vi "PIN Verification.vi"(8 "error in (no error)":errorcluster, 10 "Array":refnum<vi>[](array[refnum]), 11 "PIN in":string) -> (0 "error out":errorcluster, 1 "Right Menu":T1, 2 "Left Menu":T1, 3 "Message Out":string, 5 "PIN":string)   [LabVIEW 2019]
uses:
  controls/Read & Write File.ctl
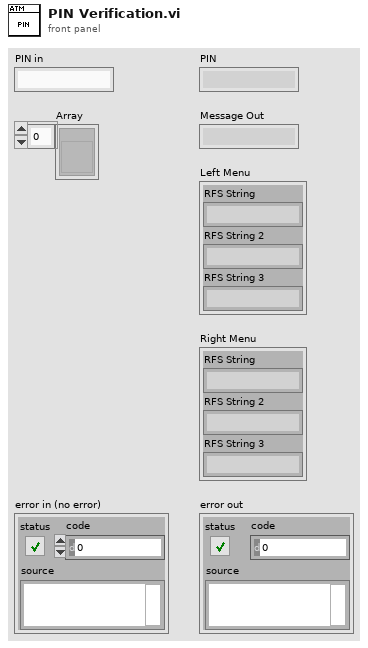
[diagram p1: front panel]
types:
  T1 = cluster{"RFS String":string, "RFS String 2":string, "RFS String 3":string}
  T2 = typedef "Read & Write File.ctl" = enum16{"Get Name", "Update Balance", "Init", "Get Balance"}
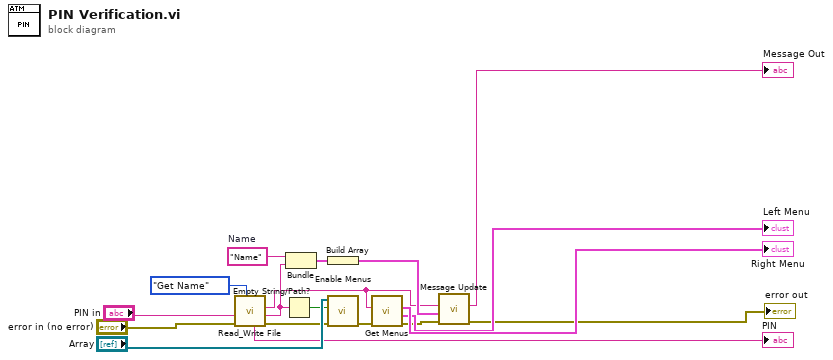
[diagram p0: block diagram]
diagram:
  w9 = "Name"  # Name
  n1 = call "Read_Write File.vi"("Read/Write File"=Read_&_Write_File."Get Name", "error in"="error in (no error)", "User Input"="PIN in") -> ("error out"=w2:errorcluster, "Output Value"=w12:string, "Message type"=w6:string, "PIN"=→"PIN":string)  [unwired: 5 in]
  n2 = Empty String/Path?(string/path=w12) -> (empty?=w5:bool)
  n3 = Bundle("Name"=w9, "Output Value"=w12) -> (w10:cluster{"Name":string, "Output Value":string})  [unwired: 1 in]
  n4 = Build Array(w10) -> (w11:cluster{"Name":string, "Output Value":string}[])
  n5 = call "Enable Menus.vi"("error in (no error)"=w2, "Valid"=w5, "Menu references"="Array") -> ("error out"=w7:errorcluster)  [unwired: 8 in]
  n6 = call "Get Menus.vi"("error in (no error)"=w7, "Message type"=w6) -> ("error out"=w8:errorcluster, "Left Menu"=→"Left Menu":T1, "Right Menu"=→"Right Menu":T1)  [unwired: 7 in]
  n7 = call "Message Update.vi"("error in (no error)"=w8, "Replace request"=w11, "Message type"=w6) -> ("error out"=→"error out":errorcluster, "Message Out"=→"Message Out":string)  [unwired: 7 in]
